vi "UHR-Fleezers Control (host) - 10.9.vi"() -> ()   [LabVIEW 2011] (continued)
            n1210 = local write "Setpoints (V)"(w1797) -> ()
            n1211 = Multiply(x=3276.7, y=w1797) -> (x*y=w1798:cluster{"Set 1":dbl, "Set 2":dbl})
            n1212 = To Word Integer(number=w1798) -> (16bit integer=w1810:cluster{"Set 1":i16, "Set 2":i16})
          }
        }
        n1213 = Unbundle By Name(w1782) -> ("Set 1"=w1781:i16, "Set 2"=w1780:i16)
        n1214 = xnode "Read/Write Control"("FPGA VI Reference In"=w1778, "error in"=w1777, "FB Setpoint Set 1"=w1781, "FB Setpoint Set 2"=w1780) -> ("error out"=w1776:errorcluster)  [unwired: 1 out]
      }
      event "Invert GI": Value Change {
        n1215 = event-data() -> ()  [unwired: 7 out]
        n1216 = xnode "Read/Write Control"("FPGA VI Reference In"=w1815, "error in"=w1813, "Invert GI"="Invert GI", "Invert GI 2"="Invert GI") -> ("error out"=w1814:errorcluster)  [unwired: 1 out]
      }
      event "Green FB Setpoint (mV)", "Green FB Gains", "Green FB On/Off", "Current When FB OFF (%)", "Green int current ON count adj": Value Change {
        n1217 = event-data() -> ()  [unwired: 7 out]
        n1218 = local read "Green FB Setpoint (mV)"() -> (w1822:dbl)
        n1219 = local read "Current When FB OFF (%)"() -> (w1825:dbl)
        n1220 = Multiply(x=w1822, y=3.2767) -> (x*y=w1821:dbl)
        n1221 = Multiply(x=w1825, y=655.35) -> (x*y=w1826:dbl)
        n1222 = To Unsigned Word Integer(number=w1826) -> (unsigned 16bit integer=w1824:u16)
        n1223 = local read "Green int current ON count adj"() -> (w1829:u32)
        n1224 = local read "Green FB Gains"() -> (w1828:T14)
        n1225 = local read "Green Laser ON/Interlacing"() -> (w1819:bool)
        n1226 = local read "Green laser mode"() -> (w1818:enum32{"Laser ON", "Laser OFF", "Interlace"})
        n1227 = local read "Green FB On/Off"() -> (w1830:bool)
        n1228 = Equal?(x=w1818, y=enum32{"Laser ON", "Laser OFF", "Interlace"}."Interlace") -> (x = y?=w1816:bool)
        n1229 = Compound Arithmetic op=AND(w1816, w1830, w1819) -> (w1820:bool)
        n1230 = xnode "Read/Write Control"("FPGA VI Reference In"=w1833, "error in"=w1832, "Green FB Setpoint"=w1821, "Green FB On/Off"=w1820, "Current Out"=w1824, "Green int current ON count adj"=w1829, "Green FB Gains"=w1828) -> ("error out"=w1831:errorcluster)  [unwired: 1 out]
      }
      event "Green laser mode", "Green Laser ON/Interlacing": Value Change {
        n1231 = event-data() -> ()  [unwired: 7 out]
        n1232 = case shown="True" "Green Laser ON/Interlacing" {
          tunnel: "Green laser mode" -> [_ w1847]
          tunnel: [enum32{"Laser ON", "Laser OFF", "Interlace"}."Laser OFF" ("Green laser mode") w1847] -> w1835
          tunnel: [FALSE w1843] -> w1834
          frame False {
          }
          frame True {
            n1233 = local read "Green FB On/Off"() -> (w1844:bool)
            n1234 = Equal?(x=w1847, y=enum32{"Laser ON", "Laser OFF", "Interlace"}."Interlace") -> (x = y?=w1845:bool)
            n1235 = And(x=w1845, y=w1844) -> (x .and. y?=w1843:bool)
          }
        }
        n1236 = xnode "Read/Write Control"("FPGA VI Reference In"=w1840, "error in"=w1838, "Operating Mode"=w1835, "Operating Mode 2"=w1835, "Green FB On/Off"=w1834) -> ("error out"=w1839:errorcluster)  [unwired: 1 out]
      }
      event "Test ttrig": Value Change {
        n1237 = event-data() -> ()  [unwired: 7 out]
        n1238 = xnode "Read/Write Control"("FPGA VI Reference In"=w1851, "error in"=w1850, "TTrig?"=TRUE) -> ("error out"=w1849:errorcluster)  [unwired: 1 out]
      }
      event "Neg. TTrig FPGA": Value Change {
        n1239 = event-data() -> ()  [unwired: 7 out]
        n1240 = xnode "Read/Write Control"("FPGA VI Reference In"=w1855, "error in"=w1854, "TTrig Negate Pos"="Neg. TTrig FPGA") -> ()  [unwired: 2 out]
      }
      event "- phase (APD 1 Gate)", "+ phase (APD 1 Gate)": Value Change {
        n1241 = event-data() -> ()  [unwired: 7 out]
        n1242 = local read "Phase Adj. (APD 1 Gate)"() -> (w1856:i16)
        n1243 = Negate(x=w1856) -> (-x=w1864:i16)
        n1244 = Select(t=w1864, s="- phase (APD 1 Gate)", f=w1856) -> (s? t:f=w1863:i16)
        n1245 = Or(x="- phase (APD 1 Gate)", y="+ phase (APD 1 Gate)") -> (x .or. y?=w1859:bool)
        n1246 = xnode "Read/Write Control"("FPGA VI Reference In"=w1866, "error in"=w1865, "Phase count adjustment (APD 1 Gate)"=w1863) -> ("FPGA VI Reference Out"=w1861:T19, "error out"=w1862:errorcluster)
        n1247 = xnode "Read/Write Control"("FPGA VI Reference In"=w1861, "error in"=w1862, "+ phase (APD 1 Gate)"=w1859) -> ("error out"=w1860:errorcluster)  [unwired: 1 out]
      }
      event "+ phase (APD 2 Gate)", "- phase (APD 2 Gate)": Value Change {
        n1248 = event-data() -> ()  [unwired: 7 out]
        n1249 = local read "Phase Adj. (APD 2 Gate)"() -> (w1867:i16)
        n1250 = Negate(x=w1867) -> (-x=w1875:i16)
        n1251 = Select(t=w1875, s="- phase (APD 2 Gate)", f=w1867) -> (s? t:f=w1874:i16)
        n1252 = Or(x="- phase (APD 2 Gate)", y="+ phase (APD 2 Gate)") -> (x .or. y?=w1870:bool)
        n1253 = xnode "Read/Write Control"("FPGA VI Reference In"=w1877, "error in"=w1876, "Phase count adjustment (APD 2 Gate)"=w1874) -> ("FPGA VI Reference Out"=w1872:T19, "error out"=w1873:errorcluster)
        n1254 = xnode "Read/Write Control"("FPGA VI Reference In"=w1872, "error in"=w1873, "+ phase (APD 2 Gate)"=w1870) -> ("error out"=w1871:errorcluster)  [unwired: 1 out]
      }
      event "Phase Adj. (APD Acq)", "+ phase (APD Acq)", "- phase (APD Acq)": Value Change {
        n1255 = event-data() -> ()  [unwired: 7 out]
        n1256 = local read "Phase Adj. (APD Acq)"() -> (w1880:i16)
        n1257 = Negate(x=w1880) -> (-x=w1886:i16)
        n1258 = Select(t=w1886, s="+ phase (APD Acq)", f=w1880) -> (s? t:f=w1885:i16)
        n1259 = Or(x="+ phase (APD Acq)", y="- phase (APD Acq)") -> (x .or. y?=w1881:bool)
        n1260 = xnode "Read/Write Control"("FPGA VI Reference In"=w1888, "error in"=w1887, "Phase Count Adjustment (APD Acq)"=w1885) -> ("FPGA VI Reference Out"=w1883:T19, "error out"=w1884:errorcluster)
        n1261 = xnode "Read/Write Control"("FPGA VI Reference In"=w1883, "error in"=w1884, "+ phase (APD Acq)"=w1881) -> ("error out"=w1882:errorcluster)  [unwired: 1 out]
      }
      event "Phase adj. (GI)", "+ phase (GI)", "- phase (GI)": Value Change {
        n1262 = event-data() -> ()  [unwired: 7 out]
        n1263 = Negate(x="Phase adj. (GI)") -> (-x=w1897:i16)
        n1264 = Select(t=w1897, s="+ phase (GI)", f="Phase adj. (GI)") -> (s? t:f=w1896:i16)
        n1265 = Or(x="+ phase (GI)", y="- phase (GI)") -> (x .or. y?=w1892:bool)
        n1266 = xnode "Read/Write Control"("FPGA VI Reference In"=w1899, "error in"=w1898, "Phase count adjustment (GI)"=w1896) -> ("FPGA VI Reference Out"=w1894:T19, "error out"=w1895:errorcluster)
        n1267 = xnode "Read/Write Control"("FPGA VI Reference In"=w1894, "error in"=w1895, "+ phase (GI)"=w1892) -> ("error out"=w1893:errorcluster)  [unwired: 1 out]
      }
      event "Phase adj. (GI) 2", "+ phase (GI) 2", "- phase (GI) 2": Value Change {
        n1268 = event-data() -> ()  [unwired: 7 out]
        n1269 = Negate(x="Phase adj. (GI) 2") -> (-x=w1908:i16)
        n1270 = Select(t=w1908, s="+ phase (GI) 2", f="Phase adj. (GI) 2") -> (s? t:f=w1907:i16)
        n1271 = Or(x="+ phase (GI) 2", y="- phase (GI) 2") -> (x .or. y?=w1903:bool)
        n1272 = xnode "Read/Write Control"("FPGA VI Reference In"=w1910, "error in"=w1909, "Phase count adjustment (GI) 2"=w1907) -> ("FPGA VI Reference Out"=w1905:T19, "error out"=w1906:errorcluster)
        n1273 = xnode "Read/Write Control"("FPGA VI Reference In"=w1905, "error in"=w1906, "+ phase (GI) 2"=w1903) -> ("error out"=w1904:errorcluster)  [unwired: 1 out]
      }
      event "Phase adj. (Green FB)", "- phase (Green FB)", "+ phase (Green FB)": Value Change {
        n1274 = event-data() -> ()  [unwired: 7 out]
        n1275 = Negate(x="Phase adj. (Green FB)") -> (-x=w1919:i16)
        n1276 = Select(t=w1919, s="+ phase (Green FB)", f="Phase adj. (Green FB)") -> (s? t:f=w1918:i16)
        n1277 = Or(x="+ phase (Green FB)", y="- phase (Green FB)") -> (x .or. y?=w1914:bool)
        n1278 = xnode "Read/Write Control"("FPGA VI Reference In"=w1921, "error in"=w1920, "Phase count adjustment (Green FB)"=w1918) -> ("FPGA VI Reference Out"=w1916:T19, "error out"=w1917:errorcluster)
        n1279 = xnode "Read/Write Control"("FPGA VI Reference In"=w1916, "error in"=w1917, "+ phase (Green FB)"=w1914) -> ("error out"=w1915:errorcluster)  [unwired: 1 out]
      }
      event "Invert APD Gate", "APD Gate ON Count", "APD Gate OFF Count", "APD Gate", "APD Integration Time (s)", "APD 1 AO Mult.", "APD 2 AO Mult.", "On one out of X cycles": Value Change {
        n1280 = event-data() -> ()  [unwired: 7 out]
        n1281 = Add(x="GI Frequency, ON count", y="GI Frequency, OFF count") -> (x+y=w1925:u32)
        n1282 = Add(x="APD Gate ON Count", y="APD Gate OFF Count") -> (x+y=w1938:u32)
        n1283 = Multiply(x="On one out of X cycles", y=w1925) -> (x*y=w1922:u32)
        "Green FB Count" <- w1922
        n1284 = Subtract(x=w1922, y="GI Frequency, ON count") -> (x-y=w1923:u32)
        n1285 = Multiply(x=w1938, y="On one out of X cycles") -> (x*y=w1937:u32)
        n1286 = Subtract(x=w1937, y="APD Gate ON Count") -> (x-y=w1936:u32)
        n1287 = local read "DMA Update Period (s)"() -> (w1939:dbl)
        n1288 = Multiply(x="APD Integration Time (s)", y=40000000.0) -> (x*y=w1944:dbl)
        n1289 = Reciprocal(x="APD Integration Time (s)") -> (1/x=→"APD Acq Rate (Hz)":dbl)
        n1290 = To Unsigned Long Integer(number=w1944) -> (unsigned 32bit integer=w1928:u32)
        "APD Int. Count" <- w1928
        n1291 = xnode "Read/Write Control"("FPGA VI Reference In"=w1948, "error in"=w1947, "Invert APD Gate"="Invert APD Gate", "APD Gate ON Count"="APD Gate ON Count", "APD Gate OFF Count"=w1936, "APD Acq Rate Count"=w1928, "APD Gate Operating Mode"="APD Gate", "APD 1 AO scale factor"="APD 1 AO Mult.", "APD 2 AO scale factor"="APD 2 AO Mult.", "Green interlace ON count"="GI Frequency, ON count", "Green interlace OFF count"=w1923, "Green interlace ON count 2"="GI Frequency, ON count", "Green interlace OFF count 2"=w1923, "Green FB Count"=w1922) -> ("error out"=w1946:errorcluster)  [unwired: 1 out]
        n1292 = Divide(x=w1939, y="APD Integration Time (s)") -> (x/y=w1942:dbl)
        n1293 = Multiply(x=2.0, y=w1942) -> (x*y=w1941:dbl)
        n1294 = local write "APD Samples/FIFO Acq."(w1942) -> ()
        n1295 = local write "APD Elements/DMA read"(w1941) -> ()
      }
      event "Number of F/B Scans (AOD)", "Scan Speed (nm/s)", "Scan BD", "Initial delta (MHz)", "Step Size (nm)", "Scan Range (nm)": Value Change {
        w2010 = 123.0  # AOM cal (nm/MHz)
        n1296 = event-data() -> ()  [unwired: 7 out]
        n1297 = local read "BD 1 Frequency 1 (MHz)"() -> (w1993:dbl)
        n1298 = local read "AOM X Cal (nm/MHz)"() -> (w1985:dbl)
        n1299 = local read "X RF Frequency Limits (MHz)"() -> (w1997:T16)
        n1300 = local read "Y RF Frequency Limits (MHz)"() -> (w1994:T16)
        n1301 = local read "BD 2 Frequency 1 (MHz)"() -> (w1999:dbl)
        n1302 = Negate(x="Scan Range (nm)") -> (-x=w1963:dbl)
        n1303 = Divide(x=w1963, y=w1985) -> (x/y=w1967:dbl)
        n1304 = Select(t=w1997, s="Scan BD", f=w1994) -> (s? t:f=w1996:T16)
        n1305 = Select(t=w1993, s="Scan BD", f=w1999) -> (s? t:f=w1998:dbl)
        n1306 = Unbundle By Name(w1996) -> ("Maximum"=w2005:dbl, "Minimum"=w2004:dbl)
        n1307 = Add(x=w1967, y=w1998) -> (x+y=w2002:dbl)
        n1308 = Divide(x=w1963, y="Step Size (nm)") -> (x/y=w1982:dbl)
        n1309 = Divide(x="Step Size (nm)", y=w1985) -> (x/y=w1991:dbl)
        n1310 = Absolute Value(x=w1982) -> (abs(x)=w1966:dbl)
        n1311 = Sign(1:w1963) -> (0:w1964:dbl)
        n1312 = In Range and Coerce(upper limit=w2005, x=w2002, lower limit=w2004) -> (coerced(x)=w2001:dbl, In Range?=w2003:bool)
        n1313 = To Unsigned Quad Integer(1:w1966) -> (0:w1981:u64)
        "Scan steps (AOD)" <- w1981
        n1314 = call "IR AOM freq to word.vi"("Frequency In (MHz)"=w1991) -> ("Frequency Word Out (double)"=w1988:dbl)
        n1315 = Multiply(x=w1964, y=w1988) -> (x*y=w1965:dbl)
        n1316 = Subtract(x=w2002, y=w2001) -> (x-y=w2000:dbl)
        n1317 = To Quad Integer(1:w1965) -> (0:w1987:i64)
        "Incr. int (AOD)" <- w1987
        n1318 = Subtract(x=w1967, y=w2000) -> (x-y=w1986:dbl)
        "Scan Range (MHz)" <- w1986
        n1319 = Select(t=w1967, s=w2003, f=w1986) -> (s? t:f=w2006:dbl)
        n1320 = Multiply(x=w1986, y=w1985) -> (x*y=w1984:dbl)
        n1321 = Decrement(x=w1981) -> (x-1=w2034:u64)
        n1322 = Negate(x=w1984) -> (-x=w1980:dbl)
        n1323 = local write "Scan Range (nm)"(w1980) -> ()
        n1324 = Divide(x=w2006, y=w2034) -> (x/y=w1990:dbl)
        "Scan Increment (MHz)" <- w1990
        n1325 = call "IR AOM freq to word.vi"("Frequency In (MHz)"=w1990) -> ("Frequency Word Out (double)"=w1989:dbl)
        n1326 = Divide(x="Step Size (nm)", y="Scan Speed (nm/s)") -> (x/y=w1977:dbl)
        n1327 = To Quad Integer(1:w1989) -> ()  [unwired: 1 out]
        n1328 = local read "Number Interlace Sets"() -> (w1961:u8)
        n1329 = local read "AI Count (ticks)"() -> (w1962:u32)
        n1330 = local read "Total Counts (ticks)"() -> (w1960:u32)
        n1331 = local read "# Samples/trap"() -> (w1992:u32)
        n1332 = Multiply(x=w1962, y=w1961) -> (x*y=w1959:u32)
        n1333 = Divide(x=w1960, y=w1959) -> (x/y=w1958:dbl)
        n1334 = Select(t=w1993, s="Scan BD", f=w1999) -> (s? t:f=w2031:dbl)
        "Initial freq. (MHz)" <- w2031
        n1335 = Add(x=w2006, y=w2031) -> (x+y=→"Final freq. (MHz)":dbl)
        n1336 = Divide(x=w1960, y=40000000.0) -> (x/y=w1976:dbl)
        n1337 = Divide(x=w1977, y=w1976) -> (x/y=w1975:dbl)
        n1338 = To Unsigned Quad Integer(1:w1975) -> (0:w1950:u64)
        n1339 = Quotient & Remainder(x=w1950, y=u64 2) -> (x-y*floor(x/y)=w1954:u64)  [unwired: 1 out]
        n1340 = Equal?(x=w1954, y=u64 0) -> (x = y?=w1952:bool)
        n1341 = Decrement(x=w1950) -> (x-1=w1951:u64)
        n1342 = Select(t=w1950, s=w1952, f=w1951) -> (s? t:f=w1949:u64)
        "Cycles/step (AOD)" <- w1949
        n1343 = xnode "Read/Write Control"("FPGA VI Reference In"=w2042, "error in"=w2041, "Scan steps"=w1981, "Number of scans"="Number of F/B Scans (AOD)", "Cycles per step"=w1949, "Scan freq.  increment"=w1987, "Scan BD"="Scan BD") -> ("error out"=w2040:errorcluster)  [unwired: 1 out]
        n1344 = Multiply(x=w1981, y=w1949) -> (x*y=w2035:u64)
        n1345 = Multiply(x=w2035, y=u64 2) -> (x*y=w1957:u64)
        n1346 = Multiply(x=w1958, y=w1957) -> (x*y=w1956:dbl)
        "Data points/scan (f/b)" <- w1956
        n1347 = Multiply(x=w1956, y="Number of F/B Scans (AOD)") -> (x*y=w2038:dbl)
        "Data points/scans" <- w2038
        n1348 = Divide(x=w2038, y=w1992) -> (x/y=→"N sets should be saved":dbl)
        n1349 = Multiply(x=w2035, y=w1976) -> (x*y=w1974:dbl)
        "Time/Scan (s) (AOD)" <- w1974
        n1350 = Select(t=w2006, s="Scan BD", f=0.0) -> (s? t:f=w2032:dbl)
        n1351 = Select(t=0.0, s="Scan BD", f=w2006) -> (s? t:f=w2028:dbl)
        n1352 = local read "BD 2 Frequency 2 (MHz)"() -> (w2024:dbl)
        n1353 = local read "BD 1 Frequency 2 (MHz)"() -> (w2027:dbl)
        n1354 = Add(x=w2028, y=w1999) -> (x+y=w2025:dbl)
        n1355 = Add(x=w1993, y=w2032) -> (x+y=w2026:dbl)
        n1356 = Multiply(x=w1974, y=2.0) -> (x*y=w1973:dbl)
        n1357 = Multiply(x=w1973, y="Number of F/B Scans (AOD)") -> (x*y=w1970:dbl)
        n1358 = Divide(x=w1970, y=60.0) -> (x/y=→"Time to Finish All (min)":dbl)
        n1359 = Add(x="Trap 2 Bead Size (nm)", y="Trap 1 Bead Size (nm)") -> (x+y=w2014:dbl)
        n1360 = Divide(x=w2014, y=2.0) -> (x/y=w2008:dbl)
        n1361 = local read "Initial delta (MHz)"() -> (w2011:dbl)
        n1362 = Subtract(x=w2025, y=w2024) -> (x-y=w2022:dbl)
        n1363 = Subtract(x=w2026, y=w2027) -> (x-y=w2023:dbl)
        n1364 = Square(x=w2022) -> (x^2=w2021:dbl)
        n1365 = Square(x=w2023) -> (x^2=w2020:dbl)
        n1366 = Add(x=w2020, y=w2021) -> (x+y=w2019:dbl)
        n1367 = Square Root(x=w2019) -> (sqrt(x)=w2018:dbl)
        "Final delta (MHz)" <- w2018
        n1368 = Multiply(x=w2010, y=w2018) -> (x*y=w2017:dbl)
        n1369 = Multiply(x=w2011, y=w2010) -> (x*y=w2009:dbl)
        n1370 = Subtract(x=w2009, y=w2008) -> (x-y=→"Initial sep (nm)":dbl)
        n1371 = Subtract(x=w2017, y=w2008) -> (x-y=→"Final sep (nm)":dbl)
      }
      event "Freq or Amp switch first", "Swap F1 and F2", "Freq switch delay", "Amp switch delay": Value Change {
        n1372 = event-data() -> ()  [unwired: 7 out]
        n1373 = local read "Freq or Amp switch first"() -> (w2043:bool)
        n1374 = local read "Amp switch delay"() -> (w2044:u16)
        n1375 = local read "Freq switch delay"() -> (w2046:u16)
        n1376 = local read "Swap F1 and F2"() -> (w2045:bool)
        n1377 = xnode "Read/Write Control"("FPGA VI Reference In"=w2049, "error in"=w2048, "Freq switch delay"=w2046, "Swap F1 and F2"=w2045, "Amp switch delay"=w2044, "Freq or Amp switch first"=w2043) -> ("error out"=w2047:errorcluster)  [unwired: 1 out]
      }
      event "Scan steps (MCL)", "Number of scans (MCL)", "Scan Range (V)\n(of steps)", "2D or 1D Scan", "N APD Samp/step", "Fast Scan Dir", "Continuous MCL Scanning", "Scan lines (y)": Value Change {
        w2051 = 32767.0 ("y")
        n1378 = event-data() -> ()  [unwired: 7 out]
        n1379 = Select(t="Scan lines (y)", s="2D or 1D Scan", f="Number of scans (MCL)") -> (s? t:f=w2056:u64)
        n1380 = Decrement(x="Scan steps (MCL)") -> (x-1=w2072:u64)
        n1381 = Divide(x="Scan Range (V)\n(of steps)", y=w2072) -> (x/y=w2071:dbl)
        "Desired Scan Incr (V)" <- w2071
        n1382 = local read "APD Integration Time (s)"() -> (w2064:dbl)
        n1383 = Multiply(x=w2071, y=w2051) -> (x*y=w2080:dbl)
        n1384 = Divide(x=w2080, y=10.0) -> (x/y=w2070:dbl)
        "Desired incr (int)" <- w2070
        n1385 = local read "Update Count (MCL)"() -> (w2076:u32)
        n1386 = Round Toward -Infinity(1:w2070) -> (0:w2079:dbl)
        n1387 = To Word Integer(number=w2079) -> (16bit integer=w2054:i16)
        "Actual Incr. int (MCL)" <- w2054
        n1388 = Multiply(x=w2064, y=40000000.0) -> (x*y=w2077:dbl)
        n1389 = Divide(x=w2077, y=w2076) -> (x/y=w2075:dbl)
        n1390 = Multiply(x=i16 10, y=w2054) -> (x*y=w2052:i16)
        n1391 = Multiply(x="N APD Samp/step", y=w2075) -> (x*y=w2074:dbl)
        "Cycles/step (MCL)" <- w2074
        n1392 = Divide(x=w2052, y=w2051) -> (x/y=→"Actual MCL Inc (V)":dbl)
        n1393 = Multiply(x="N APD Samp/step", y="Scan steps (MCL)") -> (x*y=w2066:dbl)
        n1394 = local read "APD Samples/FIFO Acq."() -> (w2063:dbl)
        n1395 = Multiply(x=w2066, y=u64 2) -> (x*y=w2065:dbl)
        "Data points/scan (f+b)" <- w2065
        n1396 = Multiply(x=w2065, y=w2056) -> (x*y=w2083:dbl)
        "Data points/scans (MCL)" <- w2083
        n1397 = Multiply(x=w2064, y=w2065) -> (x*y=w2057:dbl)
        "Time/f+b scan (s) (MCL)" <- w2057
        n1398 = Divide(x=w2083, y=w2063) -> (x/y=→"N sets should be saved (MCL)":dbl)
        n1399 = Multiply(x=w2057, y=w2056) -> (x*y=→"Total Time (s)":dbl)
        n1400 = Not(x="Fast Scan Dir") -> (.not. x?=w2061:bool)
        n1401 = xnode "Read/Write Control"("FPGA VI Reference In"=w2087, "error in"=w2086, "Scan steps (MCL)"="Scan steps (MCL)", "Number of scans (MCL)"=w2056, "Cycles per step (MCL)"=w2074, "Scan freq.  increment (MCL)"=w2054, "1D or 2D Scan?"="2D or 1D Scan", "MCL Scan Axis"=w2061, "Cont. Scan (MCL)"="Continuous MCL Scanning") -> ("error out"=w2085:errorcluster)  [unwired: 1 out]
      }
      event "Read Cal": Value Change {
        w2089 = 1000.0 ("y")
        n1402 = event-data() -> ()  [unwired: 7 out]
        n1403 = local read "Save file name"() -> (w2114:path)
        n1404 = local write "Read Cal"(FALSE ("Read Cal")) -> ()
        n1405 = Strip Path(path=w2114) -> (stripped path=w2113:path)  [unwired: 1 out]
        n1406 = Path To String(path=w2113) -> (string=w2112:string)
        n1407 = Concatenate Strings(w2112, "\\current.cal" ("string")) -> (w2110:string)
        n1408 = String To Path(string=w2110) -> (path=w2109:path)
        n1409 = Open/Create/Replace File(file path (use dialog)=w2109, operation (0:open)=T25."open", access (0:read/write)=enum16{"read/write", "read-only", "write-only"}."read-only") -> (refnum out=w2117:refnum<file>, error out=w2103:errorcluster)  [unwired: 1 in, 3 out]
        n1410 = Deny Access(4:w2103, 7:w2117) -> (0:w2102:errorcluster, 3:w2108:refnum<file>)  [unwired: 1 out]
        n1411 = Read from Binary File(5:0.0, 8:w2102, 9:T24."big-endian, network order" ("byte order (0:big-endian, network order)"), 10:-1 ("count (1)"), 11:w2108) -> (0:w2101:errorcluster, 2:w2099:dbl[], 3:w2104:refnum<file>)  [unwired: 2 out]
        n1412 = Array To Cluster(array=w2099) -> (cluster=w2098:T27)
        n1413 = Unbundle(w2098) -> ("[0]"=w2097:dbl, "[1]"=w2096:dbl, "[2]"=w2095:dbl, "[3]"=w2094:dbl, "[4]"=w2093:dbl, "[5]"=w2092:dbl)
        n1414 = Close File(refnum=w2104, error in=w2101) -> (error out=→"Read cal error":errorcluster)  [unwired: 1 out]
        n1415 = Multiply(x=w2092, y=w2089) -> (x*y=w2090:dbl)
        n1416 = local write "T2 kappa_x (pN/nm)"(w2094) -> ()
        n1417 = local write "T1 kappa_x (pN/nm)"(w2095) -> ()
        n1418 = local write "T1 alpha_x (nm/V)"(w2097) -> ()
        n1419 = local write "T2 alpha_x (nm/V)"(w2096) -> ()
        n1420 = Multiply(x=w2093, y=w2089) -> (x*y=w2091:dbl)
        n1421 = local write "T1 offset_x (mV)"(w2091) -> ()
        n1422 = local write "T2 offset_x (mV)"(w2090) -> ()
      }
      event "Abort MCL Scan": Value Change {
        n1423 = event-data() -> ()  [unwired: 7 out]
        n1424 = local write "MCL Scanning"(FALSE ("MCL Scanning")) -> ()
        n1425 = xnode "Read/Write Control"("FPGA VI Reference In"=w2122, "error in"=w2121, "Abort scan (MCL)"="Abort MCL Scan") -> ("error out"=w2120:errorcluster)  [unwired: 1 out]
      }
      event "Update Count (MCL)": Value Change {
        n1426 = event-data() -> ()  [unwired: 7 out]
        n1427 = xnode "Read/Write Control"("FPGA VI Reference In"=w2126, "error in"=w2125, "MCL count"="Update Count (MCL)") -> ("error out"=w2124:errorcluster)  [unwired: 1 out]
      }
      event "Phase adjust (MCL)", "+ phase (MCL)", "- phase (MCL)": Value Change {
        n1428 = event-data() -> ()  [unwired: 7 out]
        n1429 = Negate(x="Phase adjust (MCL)") -> (-x=w2135:i16)
        n1430 = Select(t=w2135, s="- phase (MCL)", f="Phase adjust (MCL)") -> (s? t:f=w2133:i16)
        n1431 = Or(x="- phase (MCL)", y="+ phase (MCL)") -> (x .or. y?=w2128:bool)
        n1432 = xnode "Read/Write Control"("FPGA VI Reference In"=w2137, "error in"=w2136, "Phase count adjustment (MCL)"=w2133) -> ("FPGA VI Reference Out"=w2129:T19, "error out"=w2130:errorcluster)
        n1433 = xnode "Read/Write Control"("FPGA VI Reference In"=w2129, "error in"=w2130, "+ phase (MCL)"=w2128) -> ("error out"=w2127:errorcluster)  [unwired: 1 out]
      }
      event "Abort AOD Scan": Value Change {
        n1434 = event-data() -> ()  [unwired: 7 out]
        n1435 = xnode "Read/Write Control"("FPGA VI Reference In"=w2141, "error in"=w2140, "Abort scan"="Abort AOD Scan") -> ("error out"=w2139:errorcluster)  [unwired: 1 out]
      }
      event "Continuous AOD Scanning": Value Change {
        n1436 = event-data() -> ()  [unwired: 7 out]
        n1437 = xnode "Read/Write Control"("FPGA VI Reference In"=w2145, "error in"=w2144, "Cont. Scan"="Continuous AOD Scanning") -> ("error out"=w2143:errorcluster)  [unwired: 1 out]
      }
      event "Index": Value Change {
        n1438 = event-data() -> ()  [unwired: 7 out]
        n1439 = call "Create new save file.vi"("Insert"="", "Ext"=".dat" ("string"), "Index In"="Index") -> ("Path Out"=→"Save file name":path, "Index Out"=w2146:dbl)
        "Save index" <- w2146
        n1440 = local write "Index"(w2146) -> ()
      }
      event "AO1", "AO2": Value Change {
        w2161 = 10.0 ("y")
        w2160 = 32767.0 ("y")
        n1441 = event-data() -> ()  [unwired: 7 out]
        n1442 = local read "AO2"() -> (w2159:dbl)
        n1443 = local read "AO1"() -> (w2156:dbl)
        n1444 = Multiply(x=w2156, y=w2160) -> (x*y=w2155:dbl)
        n1445 = Multiply(x=w2159, y=w2160) -> (x*y=w2158:dbl)
        n1446 = Divide(x=w2155, y=w2161) -> (x/y=w2154:dbl)
        n1447 = Divide(x=w2158, y=w2161) -> (x/y=w2157:dbl)
        n1448 = To Word Integer(number=w2154) -> (16bit integer=w2162:i16)
        n1449 = To Word Integer(number=w2157) -> (16bit integer=w2163:i16)
        n1450 = xnode "Read/Write Control"("FPGA VI Reference In"=w2153, "error in"=w2152, "AO1"=w2162, "AO2"=w2163) -> ("error out"=w2151:errorcluster)  [unwired: 1 out]
      }
      event "Inject Pump 1": Value Change {
        n1451 = event-data() -> ()  [unwired: 7 out]
        n1452 = local read "Use Harvard pumps\nfor beads (else Chemyx)"() -> (w2165:bool)
        n1453 = case shown="True" w2165 {
          tunnel: "Inject Pump 1" -> [w2169 w2207]
          tunnel: w2164 -> [_ w2208]
          frame False {
            n1454 = local read "Pump write delay (ms)"() -> (w2168:dbl)
            n1455 = local read "Chemyx Syringe Pump Serial Port"() -> (w2167:refnum<visa-resource-name>)
            n1456 = case shown="True" w2169 {
              tunnel: w2168 -> [w2175 w2189]
              tunnel: w2167 -> [w2172 w2188]
              frame False {
                n1457 = flat-sequence {
                  tunnel: w2172 -> [w2176]
                  tunnel: [w2176] -> w2173
                  tunnel: w2175 -> [_]
                  tunnel: [w2179] -> w2174
                  tunnel: w2173 -> [w2179]
                  tunnel: w2174 -> [w2180]
                  tunnel: [w2180] -> w2170
                  tunnel: [w2182] -> w2171
                  tunnel: w2170 -> [w2182]
                  tunnel: w2171 -> [w2184]
                  frame #0 {
                    n1458 = call "Write to pump.vi"("string"="enter pump1", "VISA resource name"=w2176) -> ()  [unwired: 1 out]
                  }
                  frame #1 {
                    n1459 = Wait (ms)(milliseconds to wait="Pump pause delay (ms)") -> ()  [unwired: 1 out]
                  }
                  frame #2 {
                    n1460 = call "Write to pump.vi"("string"="stop", "VISA resource name"=w2180) -> ()  [unwired: 1 out]
                  }
                  frame #3 {
                    n1461 = Wait (ms)(milliseconds to wait=u32 500) -> ()  [unwired: 1 out]
                  }
                  frame #4 {
                    n1462 = call "Write to pump.vi"("string"="stop", "VISA resource name"=w2184) -> ()  [unwired: 1 out]
                  }
                }
              }
              frame True {
                n1463 = flat-sequence {
                  tunnel: w2188 -> [w2198]
                  tunnel: w2189 -> [w2193]
                  tunnel: w2189 -> [w2200]
                  tunnel: w2188 -> [w2201]
                  tunnel: [w2201] -> w2186
                  tunnel: [w2203] -> w2187
                  tunnel: w2186 -> [w2203]
                  tunnel: w2187 -> [w2205]
                  frame #0 {
                    n1464 = local read "All Pump Parameters"() -> (w2192:T5)
                    n1465 = Unbundle By Name(w2192) -> ("Pump 1"=w2199:T28)
                    n1466 = call "Set pump parameters.vi"("Pump write delay (ms)"=w2193, "Volume (uL)"="Ch 1 Inject Volume (uL)", "Rate (uL/h)"="Ch 1 Inject Rate (ul/h)", "Units"=4.0, "Pump #"=1.0, "Pump Parameters In"=w2199, "VISA resource name"=w2198) -> ("Pump Parameters Out"=w2191:T28)  [unwired: 3 in]
                    n1467 = Bundle By Name(cluster=w2192, "Pump 1"=w2191) -> (w2190:T5)
                    n1468 = local write "All Pump Parameters"(w2190) -> ()
                  }
                  frame #1 {
                    n1469 = Wait (ms)(milliseconds to wait=w2200) -> ()  [unwired: 1 out]
                  }
                  frame #2 {
                    n1470 = call "Write to pump.vi"("string"="start", "VISA resource name"=w2201) -> ()  [unwired: 1 out]
                  }
                  frame #3 {
                    n1471 = Wait (ms)(milliseconds to wait=u32 500) -> ()  [unwired: 1 out]
                  }
                  frame #4 {
                    n1472 = call "Write to pump.vi"("string"="start", "VISA resource name"=w2205) -> ()  [unwired: 1 out]
                  }
                }
              }
            }
          }
          frame True {
            n1473 = case shown="False" w2207 {
              tunnel: w2208 -> [w2209 w2219]
              frame False {
                n1474 = flat-sequence {
                  tunnel: w2209 -> [w2211]
                  frame #0 {
                    n1475 = local write "Flushing P1"(FALSE ("Flushing P1")) -> ()
                    n1476 = Concatenate Strings("stop" ("string"), "\r") -> (w2213:string)
                    n1477 = VISA Write(VISA resource name=w2211, write buffer=w2213) -> ()  [unwired: 1 in, 3 out]
                  }
                  frame #1 {
                    n1478 = property on="Clear Volume P1" class="Bool (strict)"("Val(Sgnl)"=TRUE ("Value (Signaling)")) -> ()  [unwired: 2 in, 2 out]
                  }
                }
              }
              frame True {
                n1479 = local read "Normal Flow Rate (ul/h) P1"() -> (w2217:dbl)
                n1480 = Number To Decimal String(number=w2217) -> (decimal integer string=w2223:string)  [unwired: 1 in]
                n1481 = Concatenate Strings("irate  " ("string"), w2223, " u/h" ("string"), "\r") -> (w2221:string)
                n1482 = VISA Write(VISA resource name=w2219, write buffer=w2221) -> (VISA resource name out=w2218:refnum<visa-resource-name>)  [unwired: 1 in, 2 out]
                n1483 = Concatenate Strings("irun" ("string"), "\r") -> (w2225:string)
                n1484 = VISA Write(VISA resource name=w2218, write buffer=w2225) -> ()  [unwired: 1 in, 3 out]
              }
            }
          }
        }
      }
      event "Inject Pump 3": Value Change {
        n1485 = event-data() -> ()  [unwired: 7 out]
        n1486 = local read "Use Harvard pumps\nfor beads (else Chemyx)"() -> (w2228:bool)
        n1487 = case shown="True" w2228 {
          tunnel: "Inject Pump 3" -> [w2232 w2271]
          tunnel: w2227 -> [_ w2270]
          frame False {
            n1488 = local read "Pump write delay (ms)"() -> (w2231:dbl)
            n1489 = case shown="True" w2232 {
              tunnel: w2231 -> [w2238 w2252]
              tunnel: "Chemyx Syringe Pump Serial Port" -> [w2235 w2251]
              frame False {
                n1490 = flat-sequence {
                  tunnel: w2235 -> [w2239]
                  tunnel: [w2239] -> w2236
                  tunnel: w2238 -> [_]
                  tunnel: [w2242] -> w2237
                  tunnel: w2236 -> [w2242]
                  tunnel: w2237 -> [w2243]
                  tunnel: [w2243] -> w2233
                  tunnel: [w2245] -> w2234
                  tunnel: w2233 -> [w2245]
                  tunnel: w2234 -> [w2247]
                  frame #0 {
                    n1491 = call "Write to pump.vi"("string"="enter pump3", "VISA resource name"=w2239) -> ()  [unwired: 1 out]
                  }
                  frame #1 {
                    n1492 = local read "Pump pause delay (ms)"() -> (w2241:u32)
                    n1493 = Wait (ms)(milliseconds to wait=w2241) -> ()  [unwired: 1 out]
                  }
                  frame #2 {
                    n1494 = call "Write to pump.vi"("string"="stop", "VISA resource name"=w2243) -> ()  [unwired: 1 out]
                  }
                  frame #3 {
                    n1495 = Wait (ms)(milliseconds to wait=u32 0) -> ()  [unwired: 1 out]
                  }
                  frame #4 {
                    n1496 = call "Write to pump.vi"("string"="stop", "VISA resource name"=w2247) -> ()  [unwired: 1 out]
                  }
                }
              }
              frame True {
                n1497 = flat-sequence {
                  tunnel: w2251 -> [w2261]
                  tunnel: w2252 -> [w2256]
                  tunnel: w2252 -> [w2263]
                  tunnel: w2251 -> [w2264]
                  tunnel: [w2264] -> w2250
                  tunnel: [w2267] -> w2249
                  tunnel: w2250 -> [w2267]
                  tunnel: w2249 -> [w2268]
                  frame #0 {
                    n1498 = local read "All Pump Parameters"() -> (w2255:T5)
                    n1499 = Unbundle By Name(w2255) -> ("Pump 3"=w2262:T28)
                    n1500 = call "Set pump parameters.vi"("Pump write delay (ms)"=w2256, "Volume (uL)"="Ch 3 Inject Volume (uL)", "Rate (uL/h)"="Ch 3 Inject Rate (ul/h)", "Units"=4.0, "Pump #"=3.0, "Pump Parameters In"=w2262, "VISA resource name"=w2261) -> ("Pump Parameters Out"=w2254:T28)  [unwired: 3 in]
                    n1501 = Bundle By Name(cluster=w2255, "Pump 3"=w2254) -> (w2253:T5)
                    n1502 = local write "All Pump Parameters"(w2253) -> ()
                  }
                  frame #1 {
                    n1503 = Wait (ms)(milliseconds to wait=w2263) -> ()  [unwired: 1 out]
                  }
                  frame #2 {
                    n1504 = call "Write to pump.vi"("string"="start", "VISA resource name"=w2264) -> ()  [unwired: 1 out]
                  }
                  frame #3 {
                    n1505 = Wait (ms)(milliseconds to wait=u32 500) -> ()  [unwired: 1 out]
                  }
                  frame #4 {
                    n1506 = call "Write to pump.vi"("string"="start", "VISA resource name"=w2268) -> ()  [unwired: 1 out]
                  }
                }
              }
            }
          }
          frame True {
            n1507 = case shown="False" w2271 {
              tunnel: w2270 -> [w2272 w2279]
              frame False {
                n1508 = flat-sequence {
                  tunnel: w2272 -> [w2274]
                  frame #0 {
                    n1509 = local write "Flushing P3"(FALSE ("Flushing P3")) -> ()
                    n1510 = Concatenate Strings("stop" ("string"), "\r") -> (w2276:string)
                    n1511 = VISA Write(VISA resource name=w2274, write buffer=w2276) -> ()  [unwired: 1 in, 3 out]
                  }
                  frame #1 {
                    n1512 = property on="Clear Volume P3" class="Bool (strict)"("Val(Sgnl)"=TRUE ("Value (Signaling)")) -> ()  [unwired: 2 in, 2 out]
                  }
                }
              }
              frame True {
                n1513 = local read "Normal Flow Rate (ul/h) P3"() -> (w2280:dbl)
                n1514 = Number To Decimal String(number=w2280) -> (decimal integer string=w2286:string)  [unwired: 1 in]
                n1515 = Concatenate Strings("irate  " ("string"), w2286, " u/h" ("string"), "\r") -> (w2284:string)
                n1516 = VISA Write(VISA resource name=w2279, write buffer=w2284) -> (VISA resource name out=w2282:refnum<visa-resource-name>)  [unwired: 1 in, 2 out]
                n1517 = Concatenate Strings("irun" ("string"), "\r") -> (w2288:string)
                n1518 = VISA Write(VISA resource name=w2282, write buffer=w2288) -> ()  [unwired: 1 in, 3 out]
              }
            }
          }
        }
      }
      event "Inject Pump 2": Value Change {
        n1519 = event-data() -> ()  [unwired: 7 out]
        n1520 = local read "Pump write delay (ms)"() -> (w2292:dbl)
        n1521 = flat-sequence {
          tunnel: w2290 -> [w2305]
          tunnel: w2292 -> [w2301]
          tunnel: "Inject Pump 2" -> [_]
          tunnel: w2292 -> [w2307]
          tunnel: w2290 -> [w2308]
          frame #0 {
            n1522 = local read "All Pump Parameters"() -> (w2300:T5)
            n1523 = Multiply(x=60.0, y="Flush Center Ch Rate (ul/m)") -> (x*y=w2297:dbl)
            n1524 = Unbundle By Name(w2300) -> ("Pump 2"=w2306:T28)
            n1525 = call "Set pump parameters.vi"("Pump write delay (ms)"=w2301, "Volume (uL)"="Flush Center Ch Volume (uL)", "Rate (uL/h)"=w2297, "Units"=3.0, "Pump #"=2.0, "Pump Parameters In"=w2306, "VISA resource name"=w2305) -> ("Pump Parameters Out"=w2299:T28)  [unwired: 3 in]
            n1526 = Bundle By Name(cluster=w2300, "Pump 2"=w2299) -> (w2298:T5)
            n1527 = local write "All Pump Parameters"(w2298) -> ()
            n1528 = Add(x="Flush Center Ch Volume (uL)", y="Total Volume\nFlushed (uL)") -> (x+y=w2294:dbl)
            n1529 = local write "Total Volume\nFlushed (uL)"(w2294) -> ()
          }
          frame #1 {
            n1530 = Wait (ms)(milliseconds to wait=w2307) -> ()  [unwired: 1 out]
          }
          frame #2 {
            n1531 = call "Write to pump.vi"("string"="start", "VISA resource name"=w2308) -> ()  [unwired: 1 out]
          }
        }
        n1532 = local read "Chemyx Syringe Pump Serial Port"() -> (w2290:refnum<visa-resource-name>)
      }
      event "Sample Channel\nFlow": Value Change {
        n1533 = event-data() -> ()  [unwired: 7 out]
        n1534 = Select(t="irun" ("string"), s="Sample Channel\nFlow", f="stop" ("string")) -> (s? t:f=w2312:string)
        n1535 = Concatenate Strings(w2312, "\r") -> (w2315:string)
        n1536 = VISA Write(VISA resource name=w2310, write buffer=w2315) -> ()  [unwired: 1 in, 3 out]
      }
      event "Start Flow": Value Change {
        n1537 = event-data() -> ()  [unwired: 7 out]
        n1538 = local write "Sample Channel\nFlow"(TRUE ("Sample Channel\nFlow")) -> ()
        n1539 = local write "Start Flow"(FALSE ("Start Flow")) -> ()
        n1540 = Concatenate Strings("irun" ("string"), "\r") -> (w2321:string)
        n1541 = VISA Write(VISA resource name=w2317, write buffer=w2321) -> ()  [unwired: 1 in, 3 out]
      }
      event "Stop Flow": Value Change {
        w2323 = FALSE ("Stop Flow")
        n1542 = event-data() -> ()  [unwired: 7 out]
        n1543 = local write "Stop Flow"(w2323) -> ()
        n1544 = local write "Sample Channel\nFlow"(w2323) -> ()
        n1545 = Concatenate Strings("stop" ("string"), "\r") -> (w2326:string)
        n1546 = VISA Write(VISA resource name=w2324, write buffer=w2326) -> ()  [unwired: 1 in, 3 out]
      }
      event "Flow rate (uL/h)": Value Change {
        n1547 = event-data() -> ()  [unwired: 7 out]
        n1548 = Number To Decimal String(number="Flow rate (uL/h)") -> (decimal integer string=w2333:string)  [unwired: 1 in]
        n1549 = Concatenate Strings("irate  " ("string"), w2333, " u/h" ("string"), "\r") -> (w2332:string)
        n1550 = VISA Write(VISA resource name=w2329, write buffer=w2332) -> ()  [unwired: 1 in, 3 out]
      }
      event "Flush Sample": Value Change {
        n1551 = event-data() -> ()  [unwired: 7 out]
        n1552 = flat-sequence {
          tunnel: w2338 -> [w2366]
          tunnel: [w2346] -> w2337
          tunnel: [w2340] -> w2335
          tunnel: w2337 -> [w2370]
          tunnel: [w2370] -> w2336
          tunnel: w2335 -> [w2369]
          tunnel: w2336 -> [w2375]
          frame #0 {
            # "set paramaters (rate, volume) for flush, clear volume"
            n1553 = Number To Decimal String(number="Flush rate (uL/m)") -> (decimal integer string=w2362:string)  [unwired: 1 in]
            n1554 = Concatenate Strings("irate  " ("string"), w2362, " u/m" ("string"), "\r") -> (w2364:string)
            n1555 = VISA Write(VISA resource name=w2366, write buffer=w2364) -> (VISA resource name out=w2360:refnum<visa-resource-name>)  [unwired: 1 in, 2 out]
            n1556 = Reciprocal(x="Flush rate (uL/m)") -> (1/x=w2343:dbl)
            n1557 = Number To Decimal String(number="Volume (uL)") -> (decimal integer string=w2351:string)  [unwired: 1 in]
            n1558 = Multiply(x="Volume (uL)", y=w2343) -> (x*y=w2342:dbl)
            n1559 = Concatenate Strings("tvolume  " ("string"), w2351, " u" ("string"), "\r") -> (w2349:string)
            n1560 = Multiply(x=w2342, y=60000.0) -> (x*y=w2340:dbl)
            n1561 = VISA Write(VISA resource name=w2360, write buffer=w2349) -> (VISA resource name out=w2348:refnum<visa-resource-name>)  [unwired: 1 in, 2 out]
            n1562 = Concatenate Strings("cvolume" ("string"), "\r") -> (w2347:string)
            n1563 = VISA Write(VISA resource name=w2348, write buffer=w2347) -> (VISA resource name out=w2358:refnum<visa-resource-name>)  [unwired: 1 in, 2 out]
            n1564 = Concatenate Strings("irun" ("string"), "\r") -> (w2356:string)
            n1565 = VISA Write(VISA resource name=w2358, write buffer=w2356) -> (VISA resource name out=w2346:refnum<visa-resource-name>)  [unwired: 1 in, 2 out]
          }
          frame #1 {
            # "Have to wait until\nflow is done to reset\nrate"
            n1566 = Add(x=w2369, y=100.0) -> (x+y=w2368:dbl)
            n1567 = Wait (ms)(milliseconds to wait=w2368) -> ()  [unwired: 1 out]
          }
          frame #2 {
            # "reset flow rate to usual flow rate"
            n1568 = local read "Flow rate (uL/h)"() -> (w2381:dbl)
            n1569 = Number To Decimal String(number=w2381) -> (decimal integer string=w2379:string)  [unwired: 1 in]
            n1570 = Concatenate Strings("irate  " ("string"), w2379, " u/h" ("string"), "\r") -> (w2377:string)
            n1571 = VISA Write(VISA resource name=w2375, write buffer=w2377) -> (VISA resource name out=w2371:refnum<visa-resource-name>)  [unwired: 1 in, 2 out]
            n1572 = Concatenate Strings("cvolume" ("string"), "\r") -> (w2372:string)
            n1573 = VISA Write(VISA resource name=w2371, write buffer=w2372) -> ()  [unwired: 1 in, 3 out]
          }
        }
      }
      event "Flush Pump 3": Value Change {
        n1574 = event-data() -> ()  [unwired: 7 out]
        n1575 = flat-sequence {
          tunnel: w2382 -> [w2385]
          frame #0 {
            # "set paramaters (rate, volume) for flush, clear volume"
            n1576 = Number To Decimal String(number="Flush rate (uL/m) P3") -> (decimal integer string=w2407:string)  [unwired: 1 in]
            n1577 = local write "Inject Pump 3"(TRUE ("Inject Pump 3")) -> ()
            n1578 = Concatenate Strings("irate  " ("string"), w2407, " u/m" ("string"), "\r") -> (w2409:string)
            n1579 = VISA Write(VISA resource name=w2385, write buffer=w2409) -> (VISA resource name out=w2405:refnum<visa-resource-name>)  [unwired: 1 in, 2 out]
            n1580 = Reciprocal(x="Flush rate (uL/m) P3") -> (1/x=w2389:dbl)
            n1581 = Number To Decimal String(number="Volume (uL) P3") -> (decimal integer string=w2396:string)  [unwired: 1 in]
            n1582 = Multiply(x="Volume (uL) P3", y=w2389) -> (x*y=w2388:dbl)
            n1583 = Concatenate Strings("tvolume  " ("string"), w2396, " u" ("string"), "\r") -> (w2394:string)
            n1584 = Multiply(x=w2388, y=60.0) -> (x*y=→"HP3 Flush Time (s)":dbl)
            n1585 = VISA Write(VISA resource name=w2405, write buffer=w2394) -> (VISA resource name out=w2393:refnum<visa-resource-name>)  [unwired: 1 in, 2 out]
            n1586 = Concatenate Strings("cvolume" ("string"), "\r") -> (w2392:string)
            n1587 = VISA Write(VISA resource name=w2393, write buffer=w2392) -> (VISA resource name out=w2403:refnum<visa-resource-name>)  [unwired: 1 in, 2 out]
            n1588 = Concatenate Strings("irun" ("string"), "\r") -> (w2401:string)
            n1589 = VISA Write(VISA resource name=w2403, write buffer=w2401) -> ()  [unwired: 1 in, 3 out]
          }
          frame #1 {
            "Flushing P3" <- TRUE ("Flushing P3")
          }
        }
      }
      event "Flush Pump 1": Value Change {
        n1590 = event-data() -> ()  [unwired: 7 out]
        n1591 = flat-sequence {
          tunnel: [w2423] -> w2413
          tunnel: w2412 -> [w2416]
          tunnel: w2413 -> [_]
          frame #0 {
            # "set paramaters (rate, volume) for flush, clear volume"
            n1592 = local write "Inject Pump 1"(TRUE ("Inject Pump 1")) -> ()
            n1593 = Number To Decimal String(number="Flush rate (uL/m) P1") -> (decimal integer string=w2439:string)  [unwired: 1 in]
            n1594 = Concatenate Strings("irate  " ("string"), w2439, " u/m" ("string"), "\r") -> (w2441:string)
            n1595 = VISA Write(VISA resource name=w2416, write buffer=w2441) -> (VISA resource name out=w2437:refnum<visa-resource-name>)  [unwired: 1 in, 2 out]
            n1596 = Reciprocal(x="Flush rate (uL/m) P1") -> (1/x=w2420:dbl)
            n1597 = Number To Decimal String(number="Volume (uL) P1") -> (decimal integer string=w2428:string)  [unwired: 1 in]
            n1598 = Multiply(x="Volume (uL) P1", y=w2420) -> (x*y=w2419:dbl)
            n1599 = Concatenate Strings("tvolume  " ("string"), w2428, " u" ("string"), "\r") -> (w2426:string)
            n1600 = Multiply(x=w2419, y=60.0) -> (x*y=→"HP1 Flush Time (s)":dbl)
            n1601 = VISA Write(VISA resource name=w2437, write buffer=w2426) -> (VISA resource name out=w2425:refnum<visa-resource-name>)  [unwired: 1 in, 2 out]
            n1602 = Concatenate Strings("cvolume" ("string"), "\r") -> (w2424:string)
            n1603 = VISA Write(VISA resource name=w2425, write buffer=w2424) -> (VISA resource name out=w2435:refnum<visa-resource-name>)  [unwired: 1 in, 2 out]
            n1604 = Concatenate Strings("irun" ("string"), "\r") -> (w2433:string)
            n1605 = VISA Write(VISA resource name=w2435, write buffer=w2433) -> (VISA resource name out=w2423:refnum<visa-resource-name>)  [unwired: 1 in, 2 out]
          }
          frame #1 {
            "Flushing P1" <- TRUE ("Flushing P3")
          }
        }
      }
      event "Clear Volume": Value Change {
        n1606 = event-data() -> ()  [unwired: 7 out]
        n1607 = Concatenate Strings("cvolume" ("string"), "\r") -> (w2445:string)
        n1608 = VISA Write(VISA resource name=w2444, write buffer=w2445) -> ()  [unwired: 1 in, 3 out]
      }
      event "Clear Volume P3": Value Change {
        n1609 = event-data() -> ()  [unwired: 7 out]
        n1610 = Concatenate Strings("cvolume" ("string"), "\r") -> (w2451:string)
        n1611 = VISA Write(VISA resource name=w2450, write buffer=w2451) -> ()  [unwired: 1 in, 3 out]
        n1612 = local write "Clear Volume P3"(FALSE ("Clear Volume P3")) -> ()
      }
      event "Clear Volume P1": Value Change {
        n1613 = event-data() -> ()  [unwired: 7 out]
        n1614 = Concatenate Strings("cvolume" ("string"), "\r") -> (w2456:string)
        n1615 = local write "Clear Volume P1"(FALSE ("Clear Volume P1")) -> ()
        n1616 = VISA Write(VISA resource name=w2455, write buffer=w2456) -> ()  [unwired: 1 in, 3 out]
      }
      event "Display On P3": Value Change {
        n1617 = event-data() -> ()  [unwired: 7 out]
        n1618 = Select(t="dim 100", s="Display On P3", f="dim 0") -> (s? t:f=w2462:string)
        n1619 = Concatenate Strings(w2462, "\r") -> (w2464:string)
        n1620 = VISA Write(VISA resource name=w2459, write buffer=w2464) -> ()  [unwired: 1 in, 3 out]
      }
      event "Display On P1": Value Change {
        n1621 = event-data() -> ()  [unwired: 7 out]
        n1622 = Select(t="dim 100", s="Display On P1", f="dim 0") -> (s? t:f=w2469:string)
        n1623 = Concatenate Strings(w2469, "\r") -> (w2471:string)
        n1624 = VISA Write(VISA resource name=w2466, write buffer=w2471) -> ()  [unwired: 1 in, 3 out]
      }
      event "Retract Pump 3": Value Change {
        n1625 = event-data() -> ()  [unwired: 7 out]
        n1626 = local write "Retract Pump 3"(FALSE ("Retract Pump 3")) -> ()
        n1627 = case shown="True" "Retract Pump 3" {
          tunnel: w2473 -> [_ w2476]
          frame False {
          }
          frame True {
            n1628 = Number To Decimal String(number="Retract Rate (uL/m)") -> (decimal integer string=w2494:string)  [unwired: 1 in]
            n1629 = Concatenate Strings("wrate  " ("string"), w2494, " u/m" ("string"), "\r") -> (w2496:string)
            n1630 = VISA Write(VISA resource name=w2476, write buffer=w2496) -> (VISA resource name out=w2487:refnum<visa-resource-name>)  [unwired: 1 in, 2 out]
            n1631 = Number To Decimal String(number="Retract Vol 3 (uL)") -> (decimal integer string=w2489:string)  [unwired: 1 in]
            n1632 = Concatenate Strings("tvolume  " ("string"), w2489, " u" ("string"), "\r") -> (w2486:string)
            n1633 = VISA Write(VISA resource name=w2487, write buffer=w2486) -> (VISA resource name out=w2482:refnum<visa-resource-name>)  [unwired: 1 in, 2 out]
            n1634 = Concatenate Strings("cvolume" ("string"), "\r") -> (w2483:string)
            n1635 = VISA Write(VISA resource name=w2482, write buffer=w2483) -> (VISA resource name out=w2477:refnum<visa-resource-name>)  [unwired: 1 in, 2 out]
            n1636 = Concatenate Strings("wrun" ("string"), "\r") -> (w2478:string)
            n1637 = VISA Write(VISA resource name=w2477, write buffer=w2478) -> ()  [unwired: 1 in, 3 out]
          }
        }
      }
      event "Retract Pump 1": Value Change {
        n1638 = event-data() -> ()  [unwired: 7 out]
        n1639 = local write "Retract Pump 1"(FALSE ("Retract Pump 1")) -> ()
        n1640 = case shown="True" "Retract Pump 1" {
          tunnel: w2498 -> [_ w2503]
          frame False {
          }
          frame True {
            n1641 = local read "Retract Rate (uL/m)"() -> (w2501:dbl)
            n1642 = Number To Decimal String(number=w2501) -> (decimal integer string=w2519:string)  [unwired: 1 in]
            n1643 = Concatenate Strings("wrate  " ("string"), w2519, " u/m" ("string"), "\r") -> (w2521:string)
            n1644 = VISA Write(VISA resource name=w2503, write buffer=w2521) -> (VISA resource name out=w2513:refnum<visa-resource-name>)  [unwired: 1 in, 2 out]
            n1645 = Number To Decimal String(number="Retract Vol 1 (uL)") -> (decimal integer string=w2515:string)  [unwired: 1 in]
            n1646 = Concatenate Strings("tvolume  " ("string"), w2515, " u" ("string"), "\r") -> (w2512:string)
            n1647 = VISA Write(VISA resource name=w2513, write buffer=w2512) -> (VISA resource name out=w2509:refnum<visa-resource-name>)  [unwired: 1 in, 2 out]
            n1648 = Concatenate Strings("cvolume" ("string"), "\r") -> (w2510:string)
            n1649 = VISA Write(VISA resource name=w2509, write buffer=w2510) -> (VISA resource name out=w2504:refnum<visa-resource-name>)  [unwired: 1 in, 2 out]
            n1650 = Concatenate Strings("wrun" ("string"), "\r") -> (w2505:string)
            n1651 = VISA Write(VISA resource name=w2504, write buffer=w2505) -> ()  [unwired: 1 in, 3 out]
          }
        }
      }
      event "Flip Green Filter": Value Change {
        n1652 = event-data() -> ()  [unwired: 7 out]
        n1653 = Not(x="Flip Green Filter") -> (.not. x?=w2523:bool)
        n1654 = local write "Flip Green Filter"(w2523) -> ()
        n1655 = flat-sequence {
          tunnel: w2531 -> [w2536]
          tunnel: w2530 -> [w2535]
          tunnel: [w2533] -> w2528
          tunnel: [w2532] -> w2527
          tunnel: [w2538] -> w2526
          tunnel: w2528 -> [w2538]
          tunnel: [w2537] -> w2525
          tunnel: w2527 -> [w2537]
          tunnel: w2526 -> [w2542]
          tunnel: w2525 -> [w2541]
          tunnel: [w2540] -> w2529
          frame #0 {
            n1656 = xnode "Read/Write Control"("FPGA VI Reference In"=w2536, "error in"=w2535, "Green Filter Flipper"=TRUE) -> ("FPGA VI Reference Out"=w2533:T19, "error out"=w2532:errorcluster)
          }
          frame #1 {
            n1657 = Wait (ms)(milliseconds to wait=u32 100) -> ()  [unwired: 1 out]
          }
          frame #2 {
            n1658 = xnode "Read/Write Control"("FPGA VI Reference In"=w2542, "error in"=w2541, "Green Filter Flipper"=FALSE) -> ("error out"=w2540:errorcluster)  [unwired: 1 out]
          }
        }
      }
      event "Pump 1 contents", "Pump 3 contents": Value Change {
        n1659 = event-data() -> ()  [unwired: 7 out]
        n1660 = local read "Pump 1 contents"() -> (→"Pump 1 cont disp":string)
        n1661 = local read "Pump 3 contents"() -> (→"Pump 3 cont disp":string)
      }
      event "Reset Trap Pos. FB": Value Change {
        n1662 = event-data() -> ()  [unwired: 7 out]
        n1663 = xnode "Read/Write Control"("FPGA VI Reference In"=w2548, "error in"=w2547, "Trap Pos. FB Reset"="Reset Trap Pos. FB") -> ()  [unwired: 2 out]
      }
      event "Rem fb disp offset": Value Change {
        n1664 = event-data() -> ()  [unwired: 7 out]
        n1665 = local write "Rem fb disp offset"(FALSE ("Rem fb disp offset")) -> ()
        n1666 = local read "Mean T1 Position (nm)"() -> (w2550:dbl)
        n1667 = local read "FB Trap Pos Offset"() -> (w2551:dbl)
        n1668 = Subtract(x=w2551, y=w2550) -> (x-y=w2549:dbl)
        n1669 = local write "FB Trap Pos Offset"(w2549) -> ()
      }
      event "Threshold (nm)": Value Change {
        n1670 = event-data() -> ()  [unwired: 7 out]
        n1671 = flat-sequence {
          tunnel: w2555 -> [w2563]
          tunnel: w2554 -> [w2562]
          tunnel: [w2556] -> w2553
          tunnel: w2553 -> [w2569]
          frame #0 {
            n1672 = xnode "Read/Write Control"("FPGA VI Reference In"=w2563, "error in"=w2562) -> ("FPGA VI Reference Out"=w2559:T19, "error out"=w2558:errorcluster, "FPGA TTrig Thresh"=w2560:i64)
            n1673 = local read "Threshold stored (nm)"() -> (w2568:dbl)
            n1674 = local read "Threshold (nm)"() -> (w2556:dbl)
            n1675 = local read "AOM X Cal (nm/MHz)"() -> (w2566:dbl)
            n1676 = Subtract(x=w2556, y=w2568) -> (x-y=w2567:dbl)
            n1677 = Divide(x=w2567, y=w2566) -> (x/y=w2564:dbl)
            n1678 = call "IR AOM freq to word.vi"("Frequency In (MHz)"=w2564) -> ("Frequency Word Out (double)"=w2565:dbl)
            n1679 = To Quad Integer(1:w2565) -> (0:w2561:i64)
            n1680 = Add(x=w2560, y=w2561) -> (x+y=w2557:i64)
            n1681 = xnode "Read/Write Control"("FPGA VI Reference In"=w2559, "error in"=w2558, "FPGA TTrig Thresh"=w2557) -> ()  [unwired: 2 out]
          }
          frame #1 {
            "Threshold stored (nm)" <- w2569
          }
        }
      }
      event "FB Trig Integrate": Value Change {
        n1682 = event-data() -> ()  [unwired: 7 out]
        n1683 = local read "FB Trig Integrate"() -> (w2571:u32)
        n1684 = xnode "Read/Write Control"("FPGA VI Reference In"=w2573, "error in"=w2572, "FB Trig Integrate"=w2571) -> ("error out"=w2570:errorcluster)  [unwired: 1 out]
      }
      event "11": Value Change {
        n1685 = event-data() -> ()  [unwired: 7 out]
        n1686 = local read "11"() -> (w2574:bool)
        n1687 = case shown="True" w2574 {
          frame False {
          }
          frame True {
            n1688 = local read "Messages"() -> (w2576:string)
            n1689 = call "Update messages.vi"("Message to add"="You kicked it up to 11!", "Old message string"=w2576) -> ("New message string"=w2577:string)
            n1690 = call <vilib>:"Beep.vi"() -> ()  [unwired: 12 in]
            n1691 = local write "Messages"(w2577) -> ()
          }
        }
      }
      event "Trap Pos. FB ON": Value Change {
        n1692 = event-data() -> ()  [unwired: 7 out]
        n1693 = xnode "Read/Write Control"("FPGA VI Reference In"=w2580, "error in"=w2579, "Force feedback"="Trap Pos. FB ON") -> ()  [unwired: 2 out]
      }
      event "Remove Action Offset": Value Change {
        n1694 = event-data() -> ()  [unwired: 7 out]
        n1695 = local write "Remove Action Offset"(FALSE ("Remove Action Offset")) -> ()
        n1696 = local read "Trap Pos. FB Mult Factor"() -> (w2585:i64)
        n1697 = local read "Trap Pos FB Action"() -> (w2583:i64)
        n1698 = local read "Trap Pos. FB Offset Factor"() -> (w2581:i64)
        n1699 = Multiply(x=w2585, y=w2583) -> (x*y=w2584:i64)
        n1700 = Add(x=w2584, y=w2581) -> (x+y=w2582:i64)
        n1701 = local write "Trap Pos. FB Offset Factor"(w2582) -> ()
        n1702 = xnode "Read/Write Control"("FPGA VI Reference In"=w2588, "error in"=w2587, "Trap Pos. FB Offset Factor"=w2582) -> ()  [unwired: 2 out]
      }
      event "Remove Unwinding Offset": Value Change {
        n1703 = event-data() -> ()  [unwired: 7 out]
        n1704 = local write "Remove Unwinding Offset"(FALSE ("Remove Action Offset")) -> ()
        n1705 = local read "Trap Pos. FB Mult Factor"() -> (w2600:i64)
        n1706 = local read "Trap Pos FB Action"() -> (w2598:i64)
        n1707 = local read "Trap Pos. FB Offset Factor"() -> (w2597:i64)
        n1708 = Multiply(x=w2600, y=w2598) -> (x*y=w2599:i64)
        n1709 = local read "Trap Pos. FB Mult Factor"() -> (w2596:i64)
        n1710 = Add(x=w2599, y=w2597) -> (x+y=w2590:i64)
        n1711 = Multiply(x=32768, y="factor") -> (x*y=w2593:dbl)
        n1712 = Multiply(x=w2593, y=w2596) -> (x*y=w2595:dbl)
        n1713 = Subtract(x=w2590, y=w2595) -> (x-y=w2594:dbl)
        n1714 = To Quad Integer(1:w2594) -> (0:w2589:i64)
        n1715 = xnode "Read/Write Control"("FPGA VI Reference In"=w2603, "error in"=w2602, "Trap Pos. FB Offset Factor"=w2589) -> ()  [unwired: 2 out]
        n1716 = local write "Trap Pos. FB Offset Factor"(w2589) -> ()
      }
      event "Trap Pos. FB Range", "Trap Pos. FB Gains", "Trap Pos. FB Mult Factor", "Trap Pos. FB Offset Factor", "Trap Pos FB Negate Action", "Trap Pos FB Monitor\nT1 or T2", "Differential FB?", "Negate Diff?": Value Change {
        n1717 = event-data() -> ()  [unwired: 7 out]
        n1718 = local read "Negate Diff?"() -> (w2604:bool)
        n1719 = xnode "Read/Write Control"("FPGA VI Reference In"=w2614, "error in"=w2613, "Trap Pos. FB Range"="Trap Pos. FB Range", "Trap Pos. FB Gains"="Trap Pos. FB Gains", "Trap Pos. FB Mult Factor"="Trap Pos. FB Mult Factor", "Trap Pos. FB Offset Factor"="Trap Pos. FB Offset Factor", "Trap Pos FB Negate Action"="Trap Pos FB Negate Action", "Trap Pos FB Monitor T1 or T2"="Trap Pos FB Monitor\nT1 or T2", "AI1 X Scale"="Trap Pos. AI1 X Pre-scale", "Negate Diff?"=w2604, "Diff FB Measurement?"="Differential FB?") -> ()  [unwired: 2 out]
      }
      event "Trap Pos FB SP": Value Change {
        n1720 = event-data() -> ()  [unwired: 7 out]
        n1721 = xnode "Read/Write Control"("FPGA VI Reference In"=w2617, "error in"=w2616, "Trap Pos. FB SP"="Trap Pos FB SP") -> ()  [unwired: 2 out]
      }
      event "Set Reading to\nSetpoint": Value Change {
        # "This is the actual PID input signal"
        n1722 = event-data() -> ()  [unwired: 7 out]
